vi "Translate_ACTIVXCONTAINER.vi"(8 "error IN":errorcluster, 10 "Cle":string, 11 "XYRefnum":refnum<vi>) -> (0 "error out":errorcluster)   [LabVIEW 2013]
uses:
  Dictionnary/EnumCommandDictionnaire.ctl
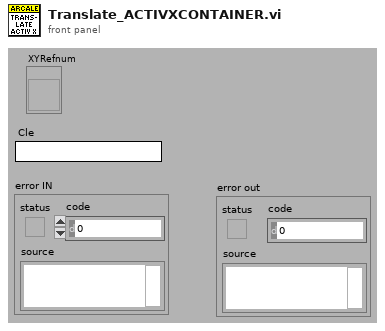
[diagram p1: front panel]
types:
  T1 = typedef "EnumCommandDictionnaire.ctl" = enum16{"Load", "Translate", "Save", "GetDico", "Set : A traduire = Vrai", "Set : A Traduire = Faux", "SetDico"}
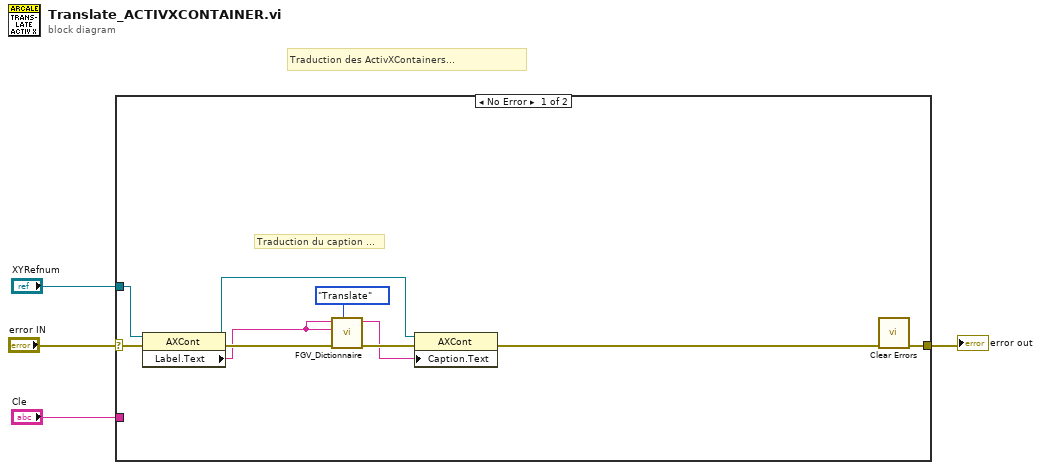
[diagram p0: block diagram]
diagram:
  # "Traduction des ActivXContainers..."
  n1 = case shown="No Error" "error IN" {
    selector: "error IN" -> [w14 w15]
    tunnel: "XYRefnum" -> [w13 _]
    tunnel: "Cle" -> [_ _]
    tunnel: [w7 w15] -> w2
    frame No Error {
      # "Traduction du caption ..."
      n2 = property class="AXCont"(reference=w13, error in=w14) -> (reference out=w12:refnum<vi>, error out=w10:errorcluster, "Label.Text"=w6:string)
      n3 = call "FGV_Dictionnaire.vi"("Command"=EnumCommandDictionnaire."Translate", "error in (no error)"=w10, "Chaîne"=w6, "Clé"=w6) -> ("error out"=w9:errorcluster, "Traduction"=w8:string)  [unwired: 5 in, 1 out]
      n4 = property class="AXCont"(reference=w12, error in=w9, "Caption.Text"=w8) -> (error out=w5:errorcluster)  [unwired: 1 out]
      n5 = call <vilib>:"Clear Errors.vi"("error in (no error)"=w5) -> ("error out"=w7:errorcluster)  [unwired: 6 in]
    }
    frame Error {
    }
  }
  "error out" <- w2
